vi "Read VIs MAP.vi"(8 "error in (no error)":errorcluster, 11 "Library in":refnum<class "Library.lvclass">) -> (0 "error out":errorcluster, 2 "VIs MAP":map{T1, refnum<class "VI.lvclass">[]}(c390), 3 "Library out":refnum<class "Library.lvclass">)   [LabVIEW 2019, in "Panther Dashboard.lvlib" / "Library.lvclass"]
uses:
  Library.lvclass
  VI/VI.lvclass
  VI Type--enum.ctl
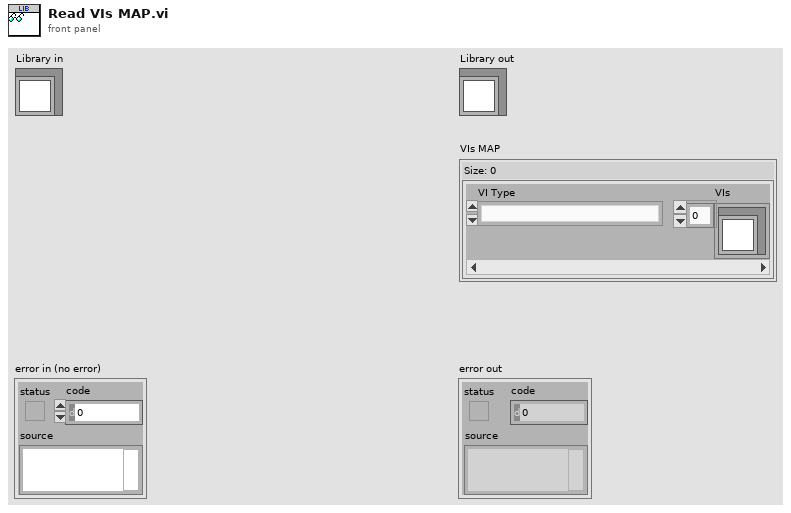
[diagram p1: front panel]
types:
  T1 = typedef "Panther Dashboard.lvlib/Library.lvclass/VI Type--enum.ctl" = enum16{"Request", "Broadcast", "Request and Wait for Reply", "Round Trip", "Public API", "Constant VI", "Error VI"}
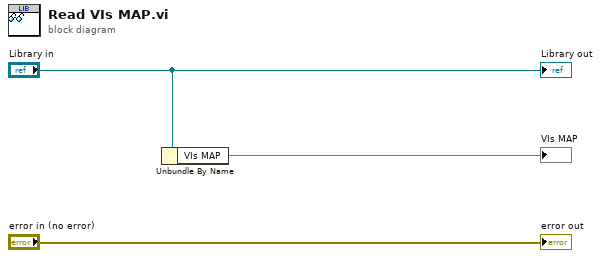
[diagram p0: block diagram]
diagram:
  n1 = Unbundle By Name("Library in") -> ("VIs MAP"=→"VIs MAP":map{T1, refnum<class "VI.lvclass">[]})
  "error out" <- "error in (no error)"
  "Library out" <- "Library in"
